vi "TRITON_PARSE_RESPONSE_FOR_NUMBER.vi"(1 "Input String":string) -> (0 "Output":dbl)   [LabVIEW 2009]
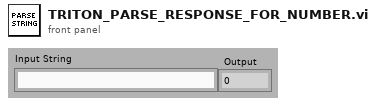
[diagram p1: front panel]
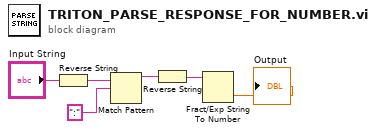
[diagram p0: block diagram]
diagram:
  n1 = Reverse String(1:"Input String") -> (0:w5:string)
  n2 = Match Pattern(string=w5, regular expression=":") -> (before substring=w3:string)  [unwired: 1 in, 3 out]
  n3 = Reverse String(1:w3) -> (0:w2:string)
  n4 = Fract/Exp String To Number(string=w2) -> (number=→"Output":dbl)  [unwired: 3 in, 1 out]
